vi "[FGV]IOParameters.vi"(7 "Enum":T3(ring)=enum."Save", 8 "error in":errorcluster, 10 "ProjectIndex":i32, 11 "DataIn":T2) -> (0 "error out":errorcluster, 2 "ProjectName":string[](array[string]), 3 "DataOut":T2)   [LabVIEW 2019]
uses:
  79c39b1a-465b-4d22-a45f-2e90e324409b.vi
  ef842f7a-5261-4f67-9249-2a75e1062a5d.vi
  GLB/IO Process GLB.vi
  <vilib>/JDP Science/JSONtext/JSON text to Variant.vi
  <vilib>/JDP Science/JSONtext/Variant to JSON Text.vi
panel:
  out "Data":T1(array[cluster])
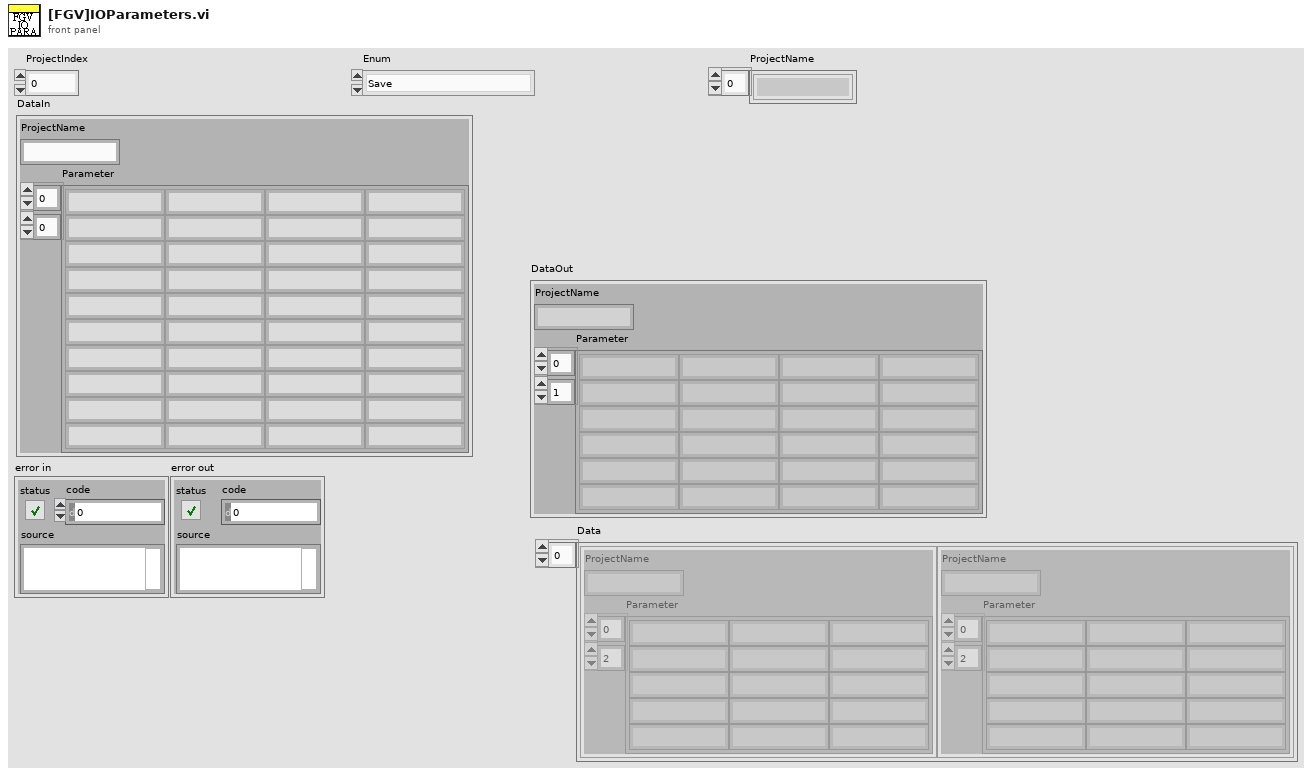
[diagram p1: front panel]
types:
  T1 = cluster{"ProjectName":string, "Parameter":string[][]}[]
  T2 = cluster{"ProjectName":string, "Parameter":string[][]}
  T3 = enum16{"initial", "write", "add", "delete", "Load", "Save", "Read", "ReadProjectName"}
  T4 = enum16{"open", "replace", "create", "open or create", "replace or create", "replace or create with confirmation"}
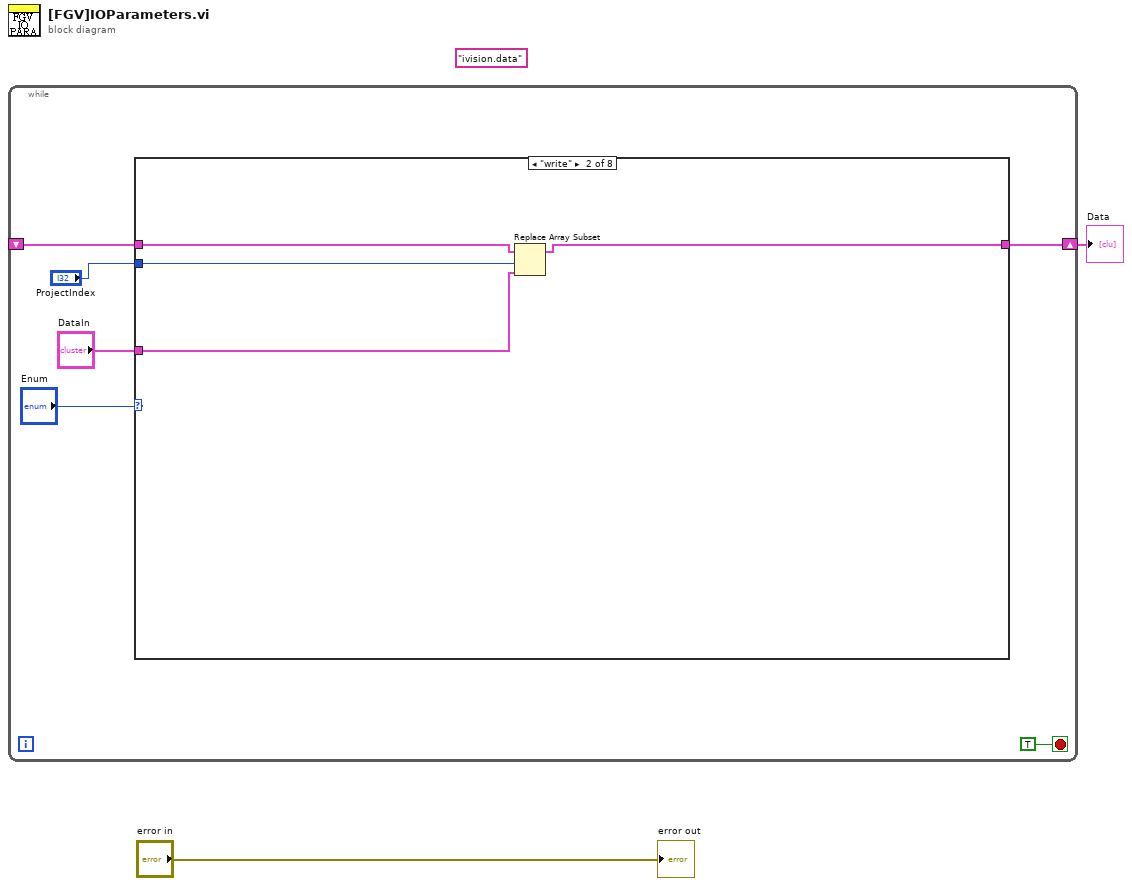
[diagram p0: block diagram]
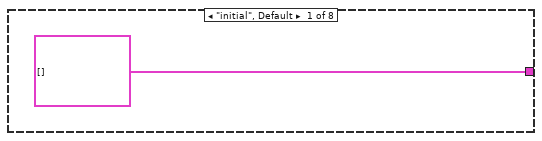
[diagram p2: hidden frame]
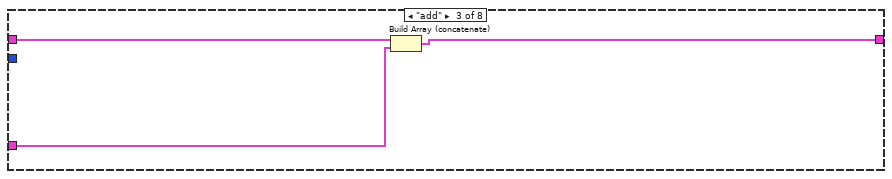
[diagram p3: hidden frame]
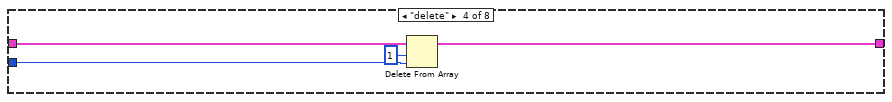
[diagram p4: hidden frame]
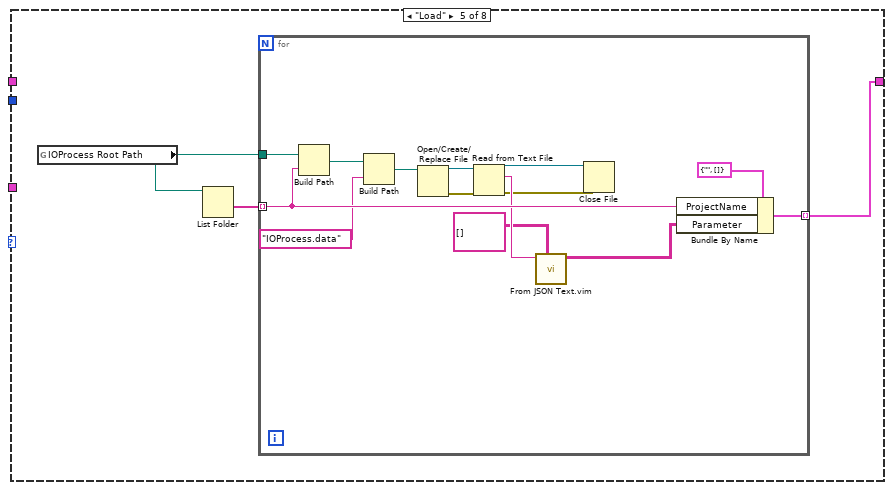
[diagram p5: hidden frame]
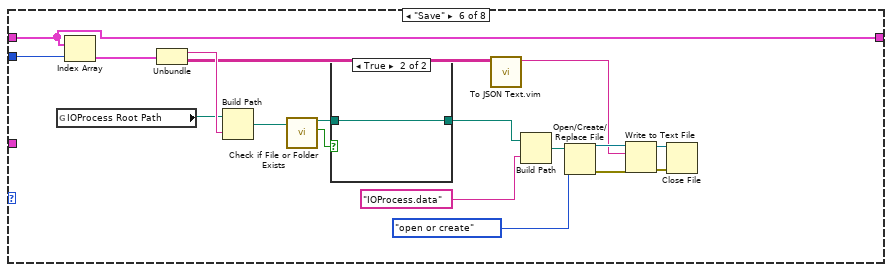
[diagram p6: hidden frame]
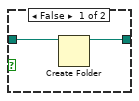
[diagram p7: hidden frame]
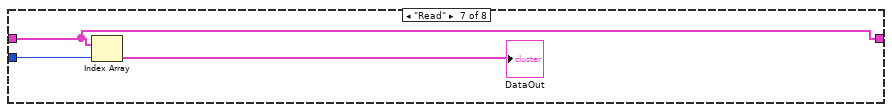
[diagram p8: hidden frame]
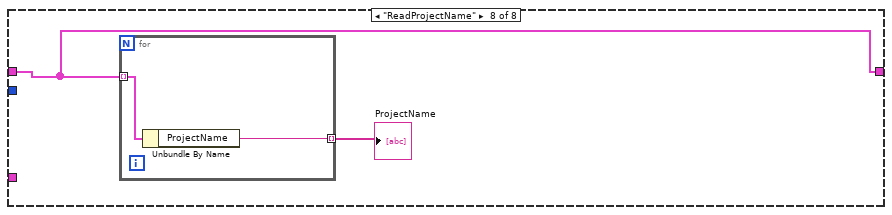
[diagram p9: hidden frame]
diagram:
  (unwired) "ivision.data" ("name or relative path")
  n1 = while {
    shift-right: [w8] -> w1
    shift-left: _ -> [w7]
    stop <- TRUE stop-if-true
    n2 = case shown="\"write\"" "Enum" {
      tunnel: [T1 [] ("Data") w12 w14 w19 w22 w54 w60 w62] -> w8
      tunnel: w7 -> [_ w13 w16 w20 _ w54 w60 w62]
      tunnel: "DataIn" -> [_ w11 w15 _ _ _ _ _]
      tunnel: "ProjectIndex" -> [_ w10 _ w18 _ w55 w61 _]
      frame "initial", Default {
      }
      frame "write" {
        n3 = Replace Array Subset(array=w13, new element=w11, index=w10) -> (w12:T1)
      }
      frame "add" {
        n4 = Build Array (concatenate)(w16, w15) -> (w14:T1)
      }
      frame "delete" {
        n5 = Delete From Array(array=w20, length=1, index=w18) -> (array with subset deleted=w19:T1)  [unwired: 1 out]
      }
      frame "Load" {
        n6 = global read "IO Process GLB.vi" "IOProcess Root Path"() -> (w21:path)
        n7 = List Folder(path=w21) -> (folder names=w23:string[])  [unwired: 3 in, 3 out]
        n8 = for {
          tunnel: w23 -> [w35] mode=indexing
          tunnel: w21 -> [w36]
          tunnel: [w24] -> w22 mode=indexing
          n9 = Build Path(base path=w36, name or relative path=w35) -> (appended path=w34:path)
          n10 = Build Path(base path=w34, name or relative path="IOProcess.data") -> (appended path=w32:path)
          n11 = Open/Create/Replace File(file path (use dialog)=w32) -> (refnum out=w30:refnum<file>, error out=w31:errorcluster)  [unwired: 5 in, 1 out]
          n12 = Read from Text File(file (use dialog)=w30, error in=w31) -> (refnum out=w28:refnum<file>, text=w29:string, error out=w27:errorcluster)  [unwired: 2 in, 1 out]
          n13 = call "From JSON Text.vim"("Data Type and Default Value"=string[][] [] ("Parameter"), "JSON"=w29) -> ("Data out"=w25:string[][])  [unwired: 8 in, 1 out]
          n14 = Close File(refnum=w28, error in=w27) -> ()  [unwired: 2 out]
          n15 = Bundle By Name(cluster=T2 {"ProjectName"="", "Parameter"=[]} ("DataIn"), "ProjectName"=w35, "Parameter"=w25) -> (w24:T2)
        }
      }
      frame "Save" {
        n16 = global read "IO Process GLB.vi" "IOProcess Root Path"() -> (w38:path)
        n17 = Index Array(array=w54, index=w55) -> (element=w53:T2)
        n18 = Unbundle(w53) -> ("ProjectName"=w52:string, "Parameter"=w42:string[][])
        n19 = Build Path(base path=w38, name or relative path=w52) -> (appended path=w51:path)
        n20 = call <vilib>:"Check if File or Folder Exists.vi"("path"=w51) -> ("file or folder exists?"=w50:bool, "dup path"=w49:path)  [unwired: 8 in, 1 out]
        n21 = case shown="True" w50 {
          tunnel: w49 -> [w57 w58]
          tunnel: [w56 w58] -> w48
          frame False {
            n22 = Create Folder(path (use dialog)=w57) -> (created path=w56:path)  [unwired: 2 in, 2 out]
          }
          frame True {
          }
        }
        n23 = call "To JSON Text.vim"("Anything"=w42) -> ("<JSON>"=w41:string)  [unwired: 9 in, 1 out]
        n24 = Build Path(base path=w48, name or relative path="IOProcess.data") -> (appended path=w46:path)
        n25 = Open/Create/Replace File(file path (use dialog)=w46, operation (0:open)=T4."open or create") -> (refnum out=w44:refnum<file>, error out=w43:errorcluster)  [unwired: 4 in, 1 out]
        n26 = Write to Text File(file (use dialog)=w44, text=w41, error in=w43) -> (refnum out=w40:refnum<file>, error out=w39:errorcluster)  [unwired: 1 in, 1 out]
        n27 = Close File(refnum=w40, error in=w39) -> ()  [unwired: 2 out]
      }
      frame "Read" {
        n28 = Index Array(array=w60, index=w61) -> (element=→"DataOut":T2)
      }
      frame "ReadProjectName" {
        n29 = for {
          tunnel: w62 -> [w65] mode=indexing
          tunnel: [w64] -> w63 mode=indexing
          n30 = Unbundle By Name(w65) -> ("ProjectName"=w64:string)
        }
        "ProjectName" <- w63
      }
    }
  }
  "Data" <- w1
  "error out" <- "error in"
